vi "Initial Values-format and values-BOOLEAN.vi"() -> (1 "Values Array":bool[](array[boolean]), 3 "Keys Array":T1)   [LabVIEW 2017]
uses:
  Typedefs/Ini file interface (Boolean).ctl
  Typedefs/HW config states enum.ctl
  Typedefs/Read Write Enum.ctl
  Global Variables/gl_UI Ctrl Refs.vi
  Global Variables/General Globals.vi
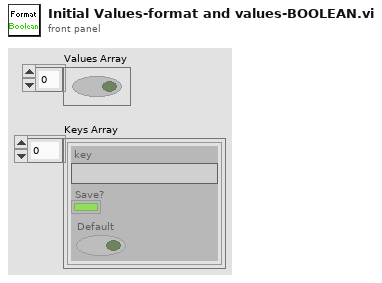
[diagram p1: front panel]
types:
  T1 = typedef "Ini file interface (Boolean).ctl" = cluster{"key":string, "Save?":bool, "Default":bool}[]
  T2 = typedef "Read Write Enum.ctl" = enum16{"Read", "Write"}
  T3 = typedef "HW config states enum.ctl" = enum16{"Load from file", "Save to file", "Write all", "Read all", "Write XY stage settings", "Write DAQ FPGA settings", "Write Control FPGA settings", "Write Phys Channels", "Write System Config", "Write HW Config", "Save System Config", "Save HW Config", "Clear", "Compare from file"}
  T4 = typedef "UI ctrl refs cluster.ctl" = cluster{"Top level VI path":path, "Top level VI ref":refnum<vi>, "User menu ref":refnum<k9>, "Sub Panel control":refnum<vi>, "Imaging Param Tab":refnum<vi>, "Occurrence-Start drivers":refnum<k4>, "Occurrence-Speed logging initialised":refnum<k4>, "Occurrence-XYZ stage initialised":refnum<k4>, "Exit button":refnum<vi>, "Status ind":refnum<vi>, "Set as origin":refnum<vi>, "Speed Logging":refnum<vi>, "Time Lapse":refnum<vi>, "Live Imaging":refnum<vi>, "AOL Z Stack":refnum<vi>, "Motor Z Stack":refnum<vi>, "Funct Acq button":refnum<vi>, "Hard Shutter":refnum<vi>, "Virtual Shutter":refnum<vi>, "Laser Power":refnum<vi>, "AOL Mode":refnum<vi>, "Frame Size":refnum<vi>, "Field of View":refnum<vi>, "Dwell Time":refnum<vi>, "Zoom":refnum<vi>, "AOL Z":refnum<vi>, "Objective":refnum<vi>, "Axis":refnum<vi>, "Paths & Names":refnum<vi>, "Experiment folder path (ind.)":refnum<vi>, "Last State (Ind.)":refnum<vi>, "Averages":refnum<vi>, "Angle (degrees)":refnum<vi>, "X centre":refnum<vi>, "Y centre":refnum<vi>, "Plane Mode":refnum<vi>, "# Planes":refnum<vi>, "Z Start":refnum<vi>, "Z Stop":refnum<vi>, "Z Step":refnum<vi>, "PMT 1":refnum<vi>, "PMT 2":refnum<vi>, "Stage XYZ Position":refnum<vi>, "Pockels@Z Start":refnum<vi>, "Pockels@Z Stop":refnum<vi>, "Obtain Z Start":refnum<vi>, "Obtain Z Stop":refnum<vi>, "Live stim.trig.period":refnum<vi>, "Live stim.trig.enable":refnum<vi>, "XY Stage Move":refnum<vi>, "Funct. Acq. Pockels Modulation":refnum<vi>, "Enable Video Recording":refnum<vi>, "Video Record-Live Imaging":refnum<vi>, "Video Record-Funct acq":refnum<vi>, "AOL Z-stack Chirps Ready (ind)":refnum<vi>, "Center freq ind (nm)":refnum<vi>, "Pickup mode (ind)":refnum<vi>, "Logging queue (ind)":refnum<vi>, "Back aperture power (ind.)":refnum<vi>, "Power after objective (ind.)":refnum<vi>, "Switch user":refnum<vi>, "Ls1 Conn. Status":refnum<vi>, "Ls1Tuning Status":refnum<vi>, "Ls1 Faults":refnum<vi>, "Ls1 Connection":refnum<vi>, "Ls1 Mode":refnum<vi>, "Ls1 POWER [mW]":refnum<vi>, "Ls1Shutter":refnum<vi>, "Ls1 Wavelength":refnum<vi>, "Ls1 Note":refnum<vi>, "Ls1 Confirm Wav":refnum<vi>, "Ls1 PreChrp Prism1":refnum<vi>, "Ls1 PreChrp Prism2":refnum<vi>, "Ls1 wav top Ind":refnum<vi>, "Ls1 power top Ind":refnum<vi>, "Ls1 Pump peak Hold":refnum<vi>, "Ls1 Status Ind":refnum<vi>, "Ls1 wav cancel":refnum<vi>, "Experiment Type":refnum<vi>, "Biology Information":refnum<vi>}
  T5 = typedef "Hardware Configuration settings.ctl" = cluster{"Dev. PC":bool, "Swap XY on stage":bool, "No of AOD":u8, "MC Supported":bool, "Axial MC":bool, "Computer MAC address":string, "Externalise Triggers":bool, "Trigger HW config":T6, "DAQmx Chan":T7, "XY stage available":bool, "XY Stage":T8, "Z stage available":bool, "Z Stage config cluster":T9, "Encoder available":bool, "Encoder":T10, "VidRec available":bool, "Cam VidRec":T11, "Laser Power Control HW config":T12, "Laser 1 available":bool, "Laser 1 config cluster":T13, "Prechirper 1 available":bool, "Prechirper 1 config cluster":T14, "Control system.FPGA available?":bool, "Control Sys. HW config":T15, "DAQ FPGA HW Config":T16}
  T6 = typedef "Triggers HW config.ctl" = cluster{"Available Device List":i32, "Device Address":string}
  T7 = typedef "DAQmx physical channels cluster.ctl" = cluster{"Pockels AO":tag, "Hard shutter AO":tag, "PMT AOs":tag, "Galvo AOs":tag, "Power meter AI":tag}
  T8 = typedef "XY Stage config cluster.ctl" = cluster{"COM port":refnum<visa-resource-name>, "Baudrate":i32, "Type":string}
  T9 = typedef "Z Stage config cluster.ctl" = cluster{"COM port":refnum<visa-resource-name>, "Baudrate":i32, "Type":string}
  T10 = typedef "Encoder config cluster.ctl" = cluster{"IP address":string, "Port":u16, "Wheel radius (cm)":dbl, "Encoder Trigger":tag}
  T11 = typedef "Cam VidRec HW config setup cluster.ctl" = cluster{"DO flag-Video record":tag, "DO flag-Trial start":tag}
  T12 = typedef "Laser Power Control HW config.ctl" = cluster{"Laser Power Control":string, "Laser Power Modulation Control":enum16{"NI", "FPGA"}}
  T13 = typedef "Laser 1 config cluster.ctl" = cluster{"COM port":refnum<visa-resource-name>, "Baud Rate":i32, "Type":string}
  T14 = typedef "PreChirper 1 config cluster.ctl" = cluster{"Type":string, "Baud Rate":i32, "COM port":refnum<visa-resource-name>}
  T15 = typedef "Control Sys HW config cluster.ctl" = cluster{"Control system.FPGA Type":enum16{"Virtex 5", "Virtex 7"}, "Control system.Network adapter name":string, "Control system.MAC address":string, "Control system.Ethernet Port":u32, "Control system.Ethernet Port Opened":bool}
  T16 = typedef "DAQ FPGA HW config cluster.ctl" = cluster{"FGPA Ref":T17, "Target":T18, "input card type":T19}
  T17 = typedef "FPGA Ref.ctl" = refnum<k20>
  T18 = typedef "nirio_resource_hc.ctl" = tag
  T19 = typedef "FPGA input type AC-DC.ctl" = enum16{"AC Card", "DC Card"}
  T20 = cluster{"key":string, "Save?":bool, "Default":bool}
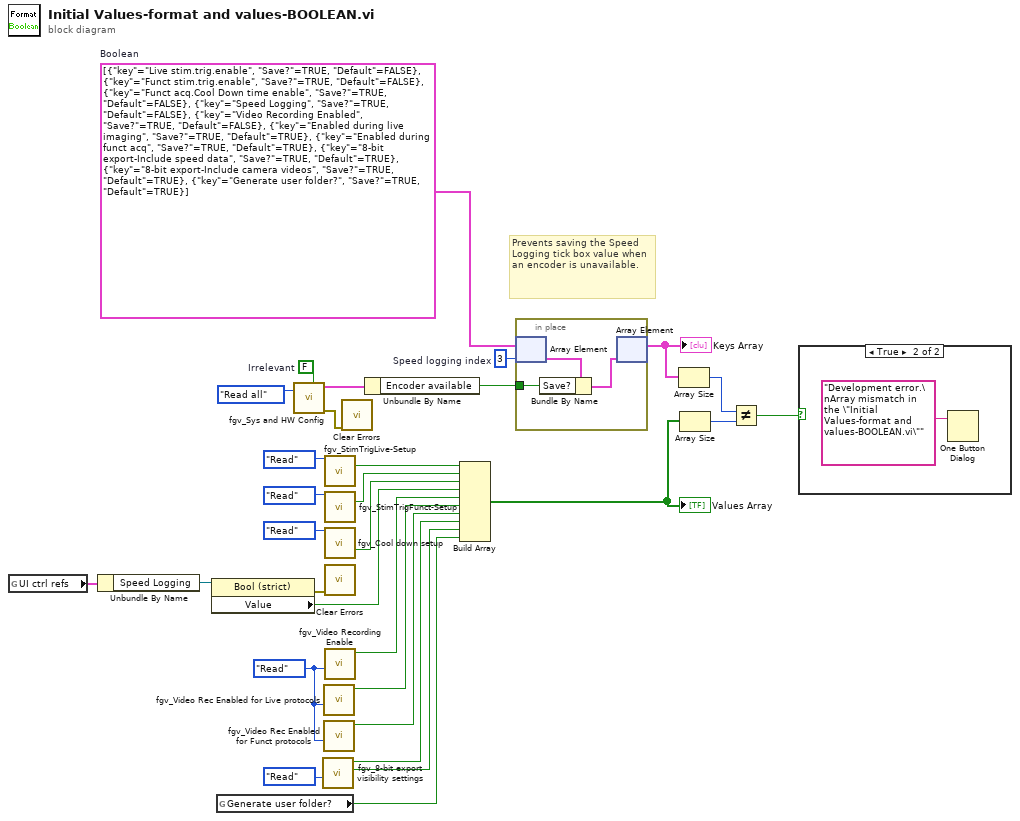
[diagram p0: block diagram]
diagram:
  w1 = FALSE  # Irrelevant
  w16 = Read_Write_Enum."Read" ("Function")
  w21 = 3  # Speed logging index
  w17 = T1 [{"key"="Live stim.trig.enable", "Save?"=TRUE, "Default"=FALSE}, {"key"="Funct stim.trig.enable", "Save?"=TRUE, "Default"=FALSE}, {"key"="Funct acq.Cool Down time enable", "Save?"=TRUE, "Default"=FALSE}, {"key"="Speed Logging", "Save?"=TRUE, "Default"=FALSE}, {"key"="Video Recording Enabled", "Save?"=TRUE, "Default"=FALSE}, {"key"="Enabled during live imaging", "Save?"=TRUE, "Default"=TRUE}, {"key"="Enabled during funct acq", "Save?"=TRUE, "Default"=TRUE}, {"key"="8-bit export-Include speed data", "Save?"=TRUE, "Default"=TRUE}, {"key"="8-bit export-Include camera videos", "Save?"=TRUE, "Default"=TRUE}, {"key"="Generate user folder?", "Save?"=TRUE, "Default"=TRUE}]  # Boolean
  # "Prevents saving the Speed Logging tick box value when an encoder is unavailable."
  n1 = global read "gl_UI Ctrl Refs.vi" "UI ctrl refs"() -> (w24:T4)
  n2 = Unbundle By Name(w24) -> ("Speed Logging"=w23:refnum<vi>)
  n3 = property class="Bool (strict)"(reference=w23) -> (error out=w4:errorcluster, "Value"=w22:bool)  [unwired: 1 in, 1 out]
  n4 = global read "General Globals.vi" "Generate user folder?"() -> (w3:bool)
  n5 = call "fgv_Sys and HW Config.vi"("Standalone viewer initialisation?"=w1, "Function"=HW_config_states_enum."Read all") -> ("error out"=w2:errorcluster, "Hardware Configuration OUT"=w20:T5)  [unwired: 7 in, 1 out]
  n6 = call "fgv_8-bit export visibility settings.vi"("Function"=enum16{"Intialize", "Write", "Read", "Clear"}."Read") -> ("Include camera videos"=w5:bool, "Include speed graph"=w6:bool)  [unwired: 8 in, 1 out]
  n7 = call "fgv_Video Rec Enabled for Live protocols.vi"("Function"=w16) -> ("Video Recording Enabled for Live protocols"=w14:bool)  [unwired: 10 in]
  n8 = call "fgv_Video Rec Enabled for Funct protocols.vi"("Function"=w16) -> ("Video Recording Enabled for functional acq protocols"=w13:bool)  [unwired: 10 in]
  n9 = call "fgv_StimTrigLive-Setup.vi"("Function"=enum16{"Intialize", "Write", "Read", "Clear"}."Read") -> ("Live stim.trig.enable"=w26:bool)  [unwired: 11 in, 3 out]
  n10 = call "fgv_StimTrigFunct-Setup.vi"("Function"=enum16{"Intialize", "Write", "Read", "Clear"}."Read") -> ("Live stim.trig.enable"=w28:bool)  [unwired: 11 in, 3 out]
  n11 = call "fgv_Cool down setup.vi"("Function"=enum16{"Intialize", "Write", "Read", "Clear"}."Read") -> ("Enable cool-down time"=w30:bool)  [unwired: 12 in, 2 out]
  n12 = call <vilib>:"Clear Errors.vi"("error in (no error)"=w4) -> ()  [unwired: 5 in, 2 out]
  n13 = call "fgv_Video Recording Enable.vi"("Function"=w16) -> ("Video Recording Enabled"=w15:bool)  [unwired: 10 in]
  n14 = call <vilib>:"Clear Errors.vi"("error in (no error)"=w2) -> ()  [unwired: 5 in, 2 out]
  n15 = Unbundle By Name(w20) -> ("Encoder available"=w18:bool)
  n16 = Build Array(w26, w28, w30, w22, w15, w14, w13, w6, w5, w3) -> (w11:bool[])
  "Values Array" <- w11
  n17 = in-place {
    in-place-border: w18 -> [w32]
    n18 = in-place-array #1(w17, w21) -> (w33:T20)
    n19 = Bundle By Name(cluster=w33, "Save?"=w32) -> (w31:T20)
    n20 = in-place-array #1(w31) -> (w12:T1)  [unwired: 1 out]
  }
  "Keys Array" <- w12
  n21 = Array Size(array=w12) -> (size(s)=w10:i32)
  n22 = Array Size(array=w11) -> (size(s)=w9:i32)
  n23 = Not Equal?(x=w10, y=w9) -> (x != y?=w8:bool)
  n24 = case shown="True" w8 {
    frame False {
    }
    frame True {
      n25 = One Button Dialog(message="Development error.\nArray mismatch in the \"Initial Values-format and values-BOOLEAN.vi\"") -> ()  [unwired: 1 in, 1 out]
    }
  }
